vi "Save_Preview.vi"() -> ()   [LabVIEW 2019]
uses:
  Control 1.ctl
  <vilib>/Utility/file.llb/Write Delimited Spreadsheet (DBL).vi
panel:
  out "Voltage Gain":i32
  out "Waveform Chart":dbl[][](graph)
  in  "file path":path=path "C:/Users/VM Lab/Desktop/labview"
  in  "Boolean":bool
  out "Data":dbl[][](array[numeric])
  out "File name":string
  out "Factor":dbl
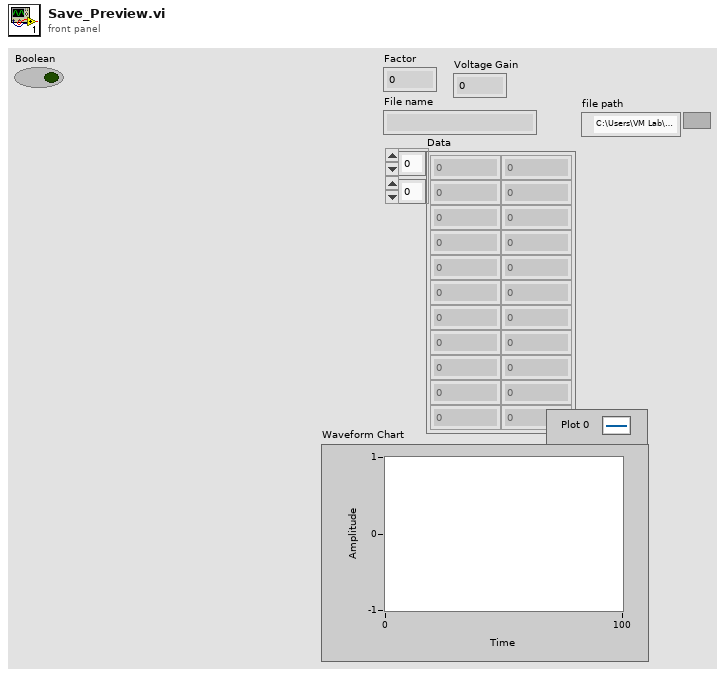
[diagram p1: front panel]
types:
  T1 = typedef "Control 1.ctl" = cluster{"Factor":dbl, "File name":string, "Data":dbl[][], "dT":dbl, "Voltage Gain":dbl}
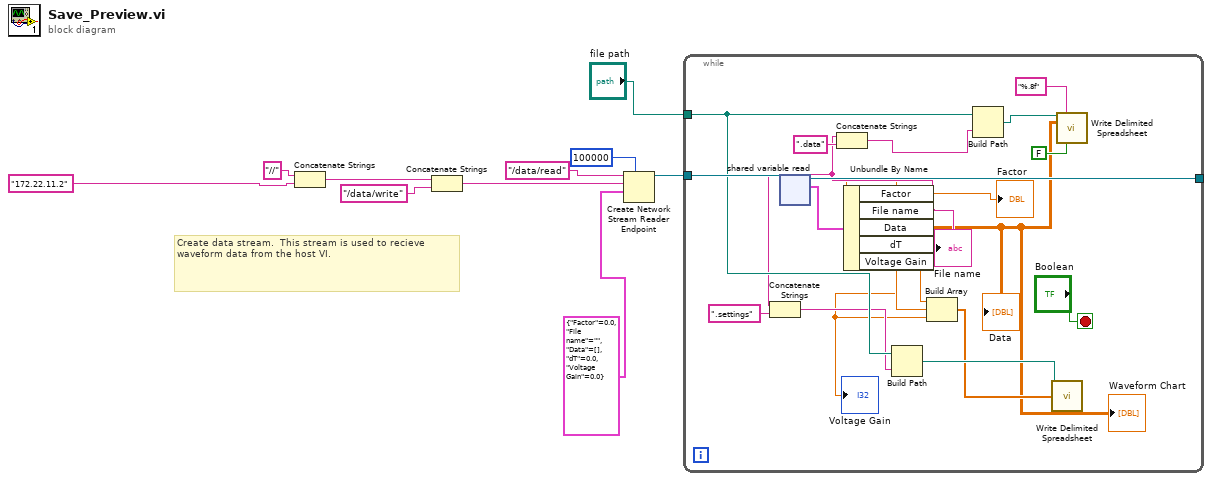
[diagram p0: block diagram]
diagram:
  # "Create data stream.  This stream is used to recieve waveform data from the host VI."
  n1 = Concatenate Strings("//" ("reader url"), "172.22.11.2" ("IP Address of cRIO")) -> (w6:string)
  n2 = Concatenate Strings(w6, "/data/write" ("reader url")) -> (w7:string)
  n3 = Create Network Stream Reader Endpoint(7:100000 ("reader buffer size"), 9:T1 {"Factor"=0.0, "File name"="", "Data"=[], "dT"=0.0, "Voltage Gain"=0.0}, 10:w7, 11:"/data/read" ("writer name")) -> (3:w2:refnum<k21>)  [unwired: 3 in, 1 out]
  n4 = while {
    tunnel: w2 -> [w29]
    tunnel: [w27] -> _
    tunnel: "file path" -> [w22]
    stop <- "Boolean" stop-if-true
    n5 = shared-variable-read(w29) -> (w27:refnum<k21>, w28:T1)  [unwired: 2 in, 2 out]
    n6 = Unbundle By Name(w28) -> ("Factor"=w14:dbl, "File name"=w18:string, "Data"=w13:dbl[][], "dT"=w16:dbl, "Voltage Gain"=w11:dbl)
    "Factor" <- w14
    "File name" <- w18
    "Data" <- w13
    "Waveform Chart" <- w13
    "Voltage Gain" <- w11
    n7 = Concatenate Strings(w18, ".settings" ("string")) -> (w19:string)
    n8 = Concatenate Strings(w18, ".data" ("string")) -> (w24:string)
    n9 = Build Path(base path=w22, name or relative path=w19) -> (appended path=w17:path)
    n10 = Build Array(w14, w16, w11) -> (w15:dbl[])
    n11 = Build Path(base path=w22, name or relative path=w24) -> (appended path=w21:path)
    n12 = call-poly <vilib>:"Write Delimited Spreadsheet.vi"("file path (dialog if empty)"=w17, "1D data"=w15) -> ()  [unwired: 12 in, 2 out]
    n13 = call-poly <vilib>:"Write Delimited Spreadsheet.vi"("file path (dialog if empty)"=w21, "format (%.3f)"="%.8f", "2D data"=w13, "transpose? (no:F)"=FALSE) -> ()  [unwired: 10 in, 2 out]
  }
